vi "Lock.vi"(8 "error in (no error)":errorcluster, 11 "B&K In":refnum<class "B&K Precision 9120 series.lvclass">) -> (0 "error out":errorcluster, 3 "B&K Out":refnum<class "B&K Precision 9120 series.lvclass">)   [LabVIEW 2014, in "B&K Precision 9120 series.lvclass"]
uses:
  B&K Precision 9120 series.lvclass
  B&K Precision 9120 series.lvclass/B&K Precision 9120 series.ctl
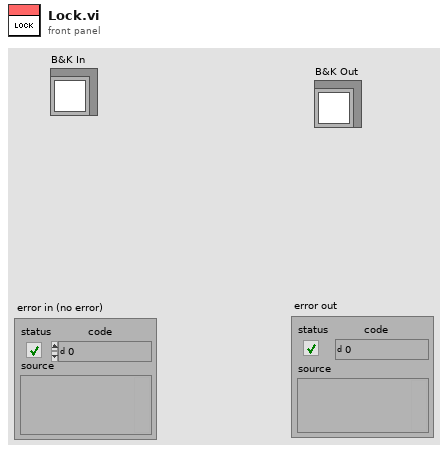
[diagram p1: front panel]
types:
  T1 = typedef "Semaphore RefNum" = refnum<k1>
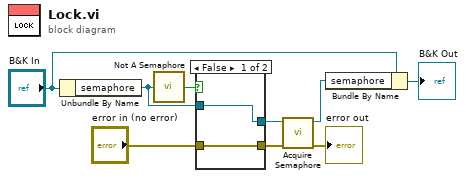
[diagram p0: block diagram]
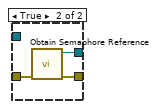
[diagram p2: hidden frame]
diagram:
  n1 = Unbundle By Name("B&K In") -> ("semaphore"=w6:T1)
  n2 = call <vilib>:"Not A Semaphore.vi"("semaphore"=w6) -> ("not a semaphore"=w7:bool)
  n3 = case shown="False" w7 {
    tunnel: [w11 w14] -> w4
    tunnel: w6 -> [w11 _]
    tunnel: "error in (no error)" -> [w10 w13]
    tunnel: [w10 w12] -> w2
    frame False {
    }
    frame True {
      n4 = call <vilib>:"Obtain Semaphore Reference.vi"("error in (no error)"=w13) -> ("error out"=w12:errorcluster, "semaphore"=w14:T1)  [unwired: 4 in, 1 out]
    }
  }
  n5 = call <vilib>:"Acquire Semaphore.vi"("error in (no error)"=w2, "semaphore"=w4) -> ("error out"=→"error out":errorcluster, "semaphore out"=w3:T1)  [unwired: 3 in, 1 out]
  n6 = Bundle By Name(cluster="B&K In", "semaphore"=w3) -> (→"B&K Out":refnum<class "B&K Precision 9120 series.lvclass">)
